vi "Force Tags Change Message DAO.vi"(8 "error in (no error)":errorcluster, 11 "DAO Actions":T1=enum."Get") -> (0 "error out":errorcluster, 2 "Force Tags":string[](array[string]), 4 "Notifier Name":string="NTCP Link Status Change")   [LabVIEW 2009]
uses:
  Data Access Objects/Metadata/DAO Actions.ctl
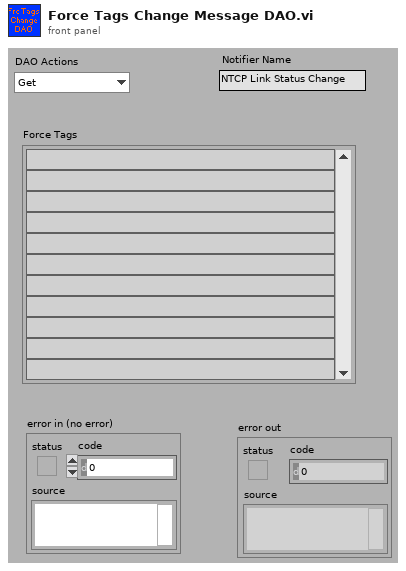
[diagram p1: front panel]
types:
  T1 = typedef "DAO Actions.ctl" = enum16{"Init", "Get", "Set"}
  T2 = typedef "Dataset Transaction Id.ctl" = cluster{"Dataset Source":T3, "Dataset Type":T4, "Hold":T5, "Volts":T5, "Tag":string}
  T3 = typedef "Dataset Source.ctl" = enum16{"LBCB 1", "LBCB 2", "Combined", "External Sensors"}
  T4 = typedef "Dataset Type.ctl" = enum16{"LVDT", "Load Cell", "Actuator Command", "Servo Error", "Displacement Command", "Displacement", "Force"}
  T5 = typedef "Yes No Button.ctl" = bool
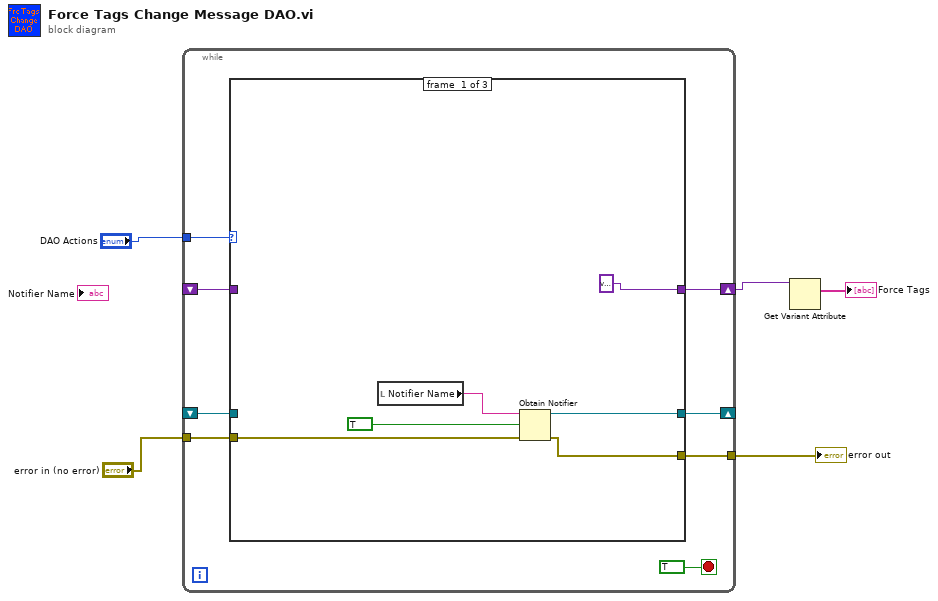
[diagram p0: block diagram]
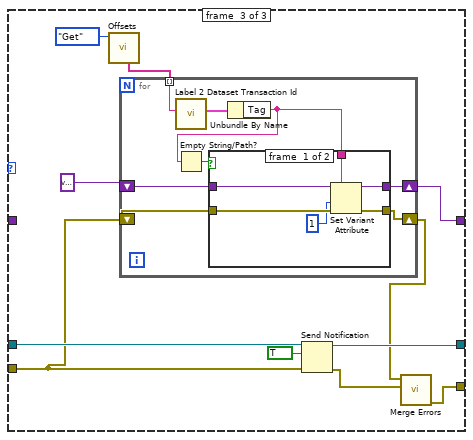
[diagram p3: hidden frame]
diagram:
  n1 = while {
    tunnel: "DAO Actions" -> [w13]
    tunnel: "error in (no error)" -> [w12]
    tunnel: [w11] -> w3
    shift-right: [w10] -> _
    shift-left: _ -> [w9]
    shift-right: [w6] -> w2
    shift-left: _ -> [w8]
    stop <- TRUE stop-if-true
    n2 = case shown="\"Set\"" w13 {
      tunnel: w12 -> [w16 w21 w26]
      tunnel: [w14 w21 w25] -> w11
      tunnel: [w17 w22 w31] -> w10
      tunnel: w9 -> [_ w22 w33]
      tunnel: w8 -> [_ w20 _]
      tunnel: [variant w20 w23] -> w6
      frame #0 {
        n3 = local read "Notifier Name"() -> (w19:string)
        n4 = Obtain Notifier(name (unnamed)=w19, notification data type=TRUE, error in (no error)=w16) -> (notifier out=w17:refnum<notifier>, error out=w14:errorcluster)  [unwired: 1 in, 1 out]
      }
      frame #1 {
      }
      frame #2 {
        n5 = call "Offsets.vi"("DAO Actions"=DAO_Actions."Get") -> ("Labels"=w28:string[])  [unwired: 8 in, 2 out]
        n6 = for {
          tunnel: w28 -> [w41] mode=indexing
          shift-right: [w39] -> w23
          shift-left: variant -> [w38]
          shift-right: [w36] -> w24
          shift-left: w26 -> [w37]
          n7 = call "Label 2 Dataset Transaction Id.vi"("Label"=w41) -> ("Dataset Trans Id"=w40:T2)  [unwired: 10 in]
          n8 = Unbundle By Name(w40) -> ("Tag"=w34:string)
          n9 = Empty String/Path?(string/path=w34) -> (empty?=w35:bool)
          n10 = case shown="False" w35 {
            tunnel: w34 -> [w47 _]
            tunnel: [w46 w49] -> w39
            tunnel: w38 -> [w45 w49]
            tunnel: w37 -> [w44 w48]
            tunnel: [w43 w48] -> w36
            frame #0 {
              n11 = Set Variant Attribute(Variant=w45, name=w47, value=1, error in=w44) -> (Variant out=w46:variant, error out=w43:errorcluster)  [unwired: 1 out]
            }
            frame #1 {
            }
          }
        }
        n12 = Send Notification(notification=TRUE, notifier=w33, error in (no error)=w26) -> (notifier out=w31:refnum<notifier>, error out=w32:errorcluster)
        n13 = call <vilib>:"Merge Errors.vi"("error in 2 (no error)"=w32, "error in 1 (no error)"=w24) -> ("error out"=w25:errorcluster)  [unwired: 5 in]
      }
    }
  }
  "error out" <- w3
  n14 = Get Variant Attribute(Variant=w2) -> (names=→"Force Tags":string[])  [unwired: 3 in, 3 out]
